vi "Voice to RGB WS2812 Control VI.vi"() -> ()   [LabVIEW 2014]
uses:
  SerialStringToRGBws28xx/VI States.ctl
  <vilib>/sound2/lvsound2.llb/Sampling Mode.ctl
  <vilib>/sound2/lvsound2.llb/Sound Data Format.ctl
  <vilib>/Analysis/baseanly.llb/Mean (DBL).vi
  <vilib>/Instr/_visa.llb/VISA Configure Serial Port (Instr).vi
  <vilib>/sound2/lvsound2.llb/Sound Input Read (DBL).vi
  <vilib>/measure/madcrms.llb/Basic Averaged DC-RMS for N Chan.vi
  <vilib>/measure/NI_MAPro.lvlib
  <vilib>/Analysis/NI_AALBase.lvlib
panel:
  in  "Start Button":bool
  in  "Device ID":u32 format="%.0x"
  in  "Number of Samples/ch":i32=5000
  in  "Stop Button":bool
  in  "VISA resource name":refnum<visa-resource-name>
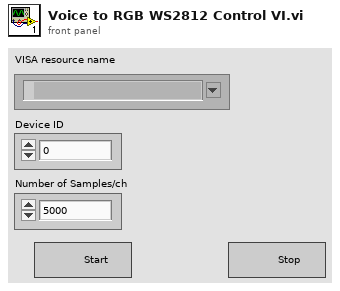
[diagram p1: front panel]
types:
  T1 = typedef "VI States.ctl" = enum16{"Poll", "Init Serial", "Read Serial", "Acq Sound", "Close Serial"}
  T2 = typedef "Sound Data Format.ctl" = cluster{"sample rate (S/s)":dbl, "number of channels":i32, "bits per sample":i32}
  T3 = typedef "Sampling Mode.ctl" = i32
  T4 = typedef "Sound Input Task ID.ctl" = u32
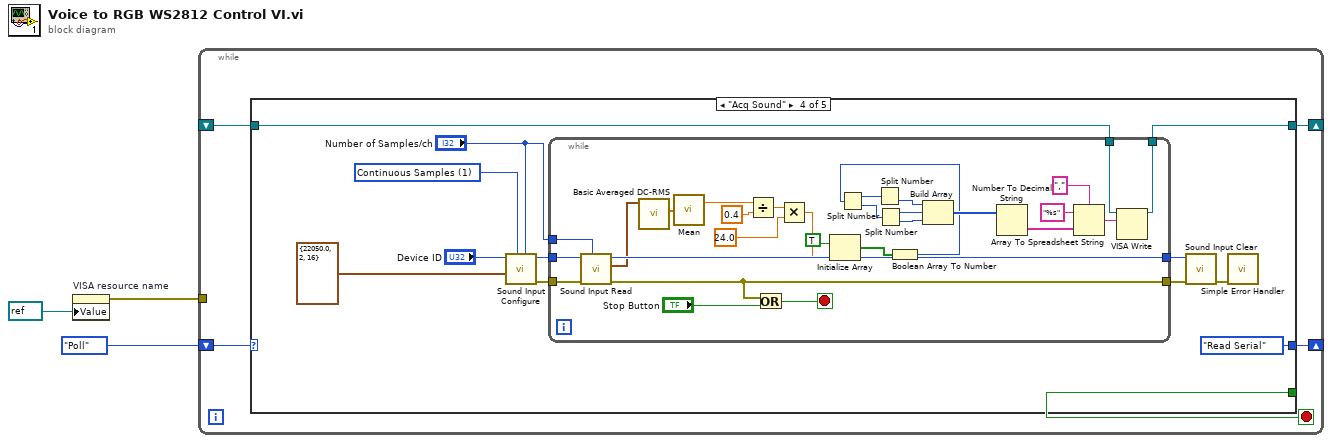
[diagram p0: block diagram]
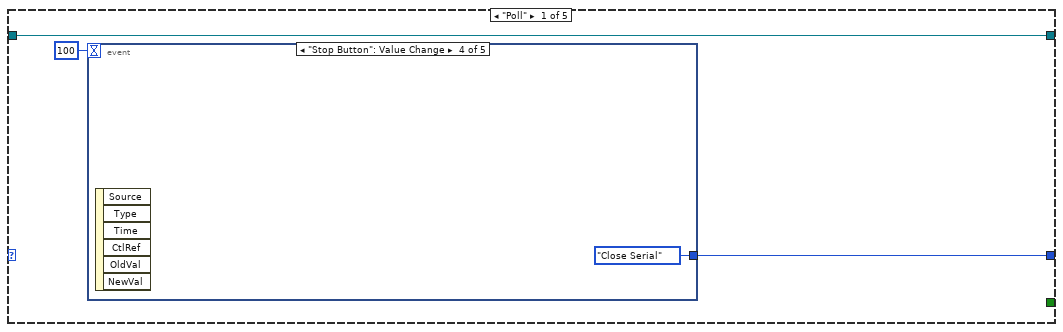
[diagram p2: hidden frame]
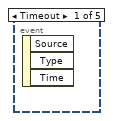
[diagram p3: hidden frame]
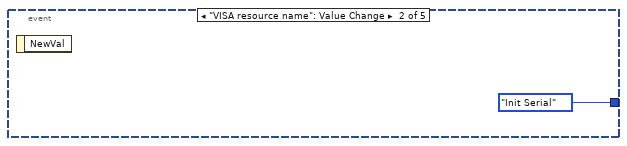
[diagram p4: hidden frame]
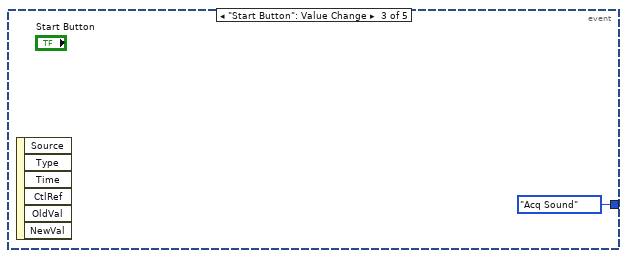
[diagram p5: hidden frame]
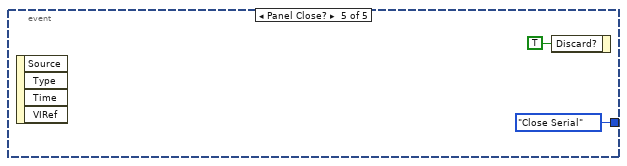
[diagram p6: hidden frame]
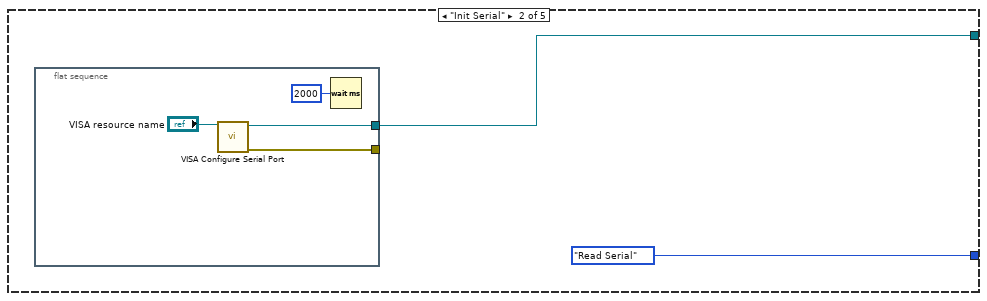
[diagram p7: hidden frame]
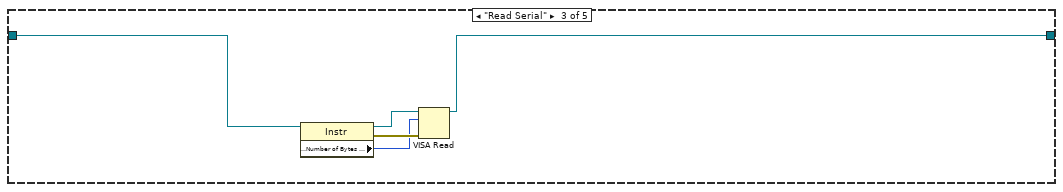
[diagram p8: hidden frame]
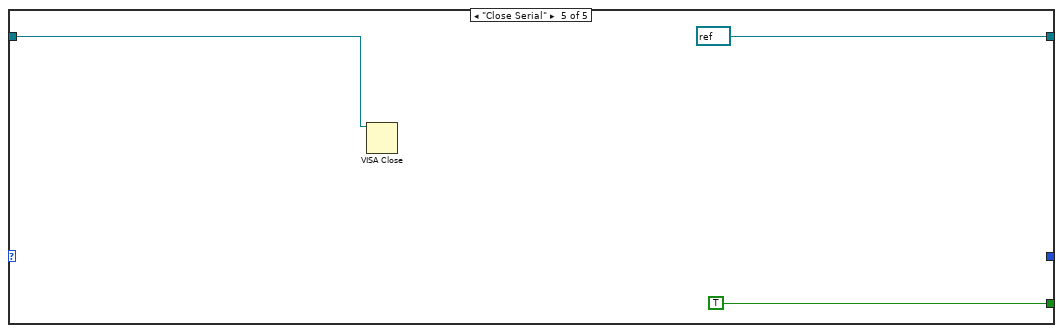
[diagram p9: hidden frame]
diagram:
  n1 = property on="VISA resource name" class="VISAName"("Value"=refnum<visa-resource-name> refnum ("VISA resource name")) -> (error out=w1:errorcluster)  [unwired: 2 in, 1 out]
  n2 = while {
    shift-right: [w7] -> _
    shift-left: VI_States."Poll" -> [w8]
    shift-right: [w6] -> _
    shift-left: _ -> [w5]
    tunnel: w1 -> [_]
    stop <- w4 stop-if-true
    n3 = case shown="\"Acq Sound\"" w8 {
      tunnel: [w10 VI_States."Read Serial" _ VI_States."Read Serial" _] -> w7
      tunnel: [w9 w18 w23 w28 refnum<visa-resource-name> refnum ("VISA resource name out")] -> w6
      tunnel: w5 -> [w9 _ w24 w29 w71]
      tunnel: [_ _ _ _ TRUE] -> w4
      frame "Poll" {
        n4 = event shown="[3] \"Stop Button\": Value Change" {
          selector: _ -> [_ _ _ _ _]
          dyn-events: _ -> [_ _ _ _ _]
          timeout: 100 -> [_ _ _ _ _]
          tunnel: [_ VI_States."Init Serial" VI_States."Acq Sound" VI_States."Close Serial" VI_States."Close Serial"] -> w10
          event Timeout {
            n5 = event-data() -> ()  [unwired: 1 in, 3 out]
          }
          event "VISA resource name": Value Change {
            n6 = event-data() -> ()  [unwired: 1 in, 1 out]
          }
          event "Start Button": Value Change {
            n7 = event-data() -> ()  [unwired: 1 in, 6 out]
          }
          event "Stop Button": Value Change {
            n8 = event-data() -> ()  [unwired: 1 in, 6 out]
          }
          event Panel Close? {
            n9 = event-data() -> ()  [unwired: 1 in, 4 out]
            n10 = event-data("Discard?"=TRUE) -> ()  [unwired: 1 in, 1 out]
          }
        }
      }
      frame "Init Serial" {
        n11 = flat-sequence {
          tunnel: [w22] -> w18
          tunnel: [w21] -> _
          frame #0 {
            n12 = call-poly "VISA Configure Serial Port"("VISA resource name"="VISA resource name") -> ("VISA resource name out"=w22:refnum<visa-resource-name>, "error out"=w21:errorcluster)  [unwired: 8 in, 5 out]
            n13 = Wait (ms)(milliseconds to wait=u32 2000) -> ()  [unwired: 1 out]
          }
        }
      }
      frame "Read Serial" {
        n14 = property class="Instr"(reference=w24) -> (reference out=w27:refnum<visa-resource-name>, error out=w26:errorcluster, "Serial Settings:Number of Bytes at Serial Port"=w25:u32)  [unwired: 1 in]
        n15 = VISA Read(VISA resource name=w27, byte count=w25, error in (no error)=w26) -> (VISA resource name out=w23:refnum<visa-resource-name>)  [unwired: 3 out]
      }
      frame "Acq Sound" {
        w35 = T3 1 items=["Finite Samples", "Continuous Samples"] ("sample mode")
        n16 = call <vilib>:"Sound Input Configure.vi"("number of samples/ch"="Number of Samples/ch", "sample mode"=w35, "sound format"=T2 {"sample rate (S/s)"=22050.0, "number of channels"=2, "bits per sample"=16} ("Sound Format"), "device ID"="Device ID") -> ("error out"=w30:errorcluster, "task ID"=w32:T4)  [unwired: 6 in]
        n17 = while {
          tunnel: w32 -> [w67]
          tunnel: [w66] -> w33
          tunnel: "Number of Samples/ch" -> [w65]
          tunnel: w30 -> [w68]
          tunnel: [w63] -> w34
          tunnel: w29 -> [w47]
          tunnel: [w46] -> w28
          stop <- w64 stop-if-true
          # "Read Sound Data"
          n18 = call-poly <vilib>:"Sound Input Read.vi"("number of samples/ch"=w65, "error in (no error)"=w68, "task ID"=w67) -> ("error out"=w63:errorcluster, "data"=w62:waveform(dbl)[], "task ID out"=w66:T4)  [unwired: 6 in]
          n19 = call-poly <vilib>:"Basic Averaged DC-RMS.vi"("signals in"=w62) -> ("RMS values"=w61:dbl[])  [unwired: 7 in, 3 out]
          n20 = call-poly <vilib>:"Mean.vi"("X"=w61) -> ("mean"=w59:dbl)  [unwired: 1 out]
          n21 = Divide(x=w59, y=0.4 ("x")) -> (x/y=w42:dbl)
          n22 = Or(x=w63, y="Stop Button") -> (x .or. y?=w64:bool)
          n23 = Multiply(x=w42, y=24.0) -> (x*y=w41:dbl)
          n24 = Initialize Array(TRUE, w41) -> (w44:bool[])
          n25 = Boolean Array To Number(Boolean array=w44) -> (number=w43:u32)
          n26 = Split Number(x=w43) -> (hi(x)=w48:u16, lo(x)=w49:u16)
          n27 = Split Number(x=w48) -> (lo(x)=w50:u8)  [unwired: 1 out]
          n28 = Split Number(x=w49) -> (hi(x)=w51:u8, lo(x)=w52:u8)
          n29 = Build Array(w50, w51, w52) -> (w57:u8[])
          n30 = Number To Decimal String(number=w57) -> (decimal integer string=w56:string[])  [unwired: 1 in]
          n31 = Array To Spreadsheet String(delimiter (Tab)=",", array=w56, 3:"%s" ("format string")) -> (spreadsheet string=w55:string)
          n32 = VISA Write(VISA resource name=w47, write buffer=w55) -> (VISA resource name out=w46:refnum<visa-resource-name>)  [unwired: 1 in, 2 out]
        }
        n33 = call <vilib>:"Sound Input Clear.vi"("error in (no error)"=w34, "task ID"=w33) -> ("error out"=w37:errorcluster)  [unwired: 9 in]
        n34 = call <vilib>:"Simple Error Handler.vi"("error in (no error)"=w37) -> ()  [unwired: 4 in, 5 out]
      }
      frame "Close Serial" {
        n35 = VISA Close(VISA resource name=w71) -> ()  [unwired: 1 in, 1 out]
      }
    }
  }
